vi "EngineUI.vi"() -> ()   [LabVIEW 2025, in "Abstract Engine.lvlib" / "Abstract Engine.lvclass"]
doc: "Copyright 2017 National Instruments Corporation\n\nLicensed under the Apache License, Version 2.0 (the \"License\"); you may not use this file except in compliance with the License. You may obtain a copy of the License at http://www.apache.org/licenses/LICENSE-2.0\nUnless required by applicable law or agreed to in writing, software distributed under the License is distributed on an \"AS IS\" BASIS, WITHOUT WARRANTIES OR CONDITIONS OF ANY KIND, either express or implied. See the License for the specific language governing permissions and limitations under the License."
uses:
  Abstract Engine.lvclass
  Abstract Engine.lvclass/Abstract Engine.ctl
  Engine configuration/Engine configuration.lvclass
  Users/Public/Documents/Sandia National Labs/TSS Plugin/CEF.lvlibp/Node/CEF_Node.lvclass
  <vilib>/Utility/sysdir.llb/System Directory Type.ctl
  Engine configuration/Engine Setting.ctl
  Users/Public/Documents/Sandia National Labs/TSS Plugin/CEF.lvlibp/Node/mainQref.ctl
  Users/Public/Documents/Sandia National Labs/TSS Plugin/CEF.lvlibp/Node/NodeRef.ctl
  Users/Public/Documents/Sandia National Labs/TSS Plugin/CEF.lvlibp/Node/UserEventRef.ctl
panel:
  in  "Engine Default":T1={"Enabled"=TRUE, "IP Address"="127.0.0.1", "Port"=3331, "Description"="Type = Class \n", "Type"="Engine", "Version"="1.0.0.0"}
  in  "user event":T2
  in  "main queue":T3
  in  "node ref":T4
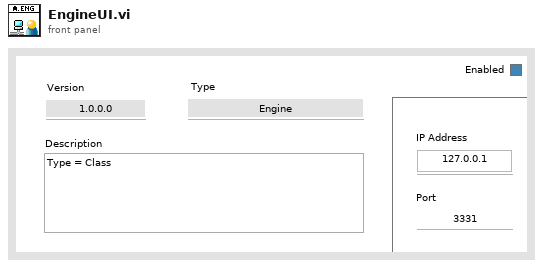
[diagram p1: front panel]
types:
  T1 = typedef "Abstract Engine.lvlib/Engine configuration.lvclass/Engine Setting.ctl" = cluster{"Enabled":bool, "IP Address":string, "Port":i32, "Description":string, "Type":string, "Version":string}
  T2 = typedef "CEF.lvlibp/CEF_Node.lvclass/UserEventRef.ctl" = refnum<user-event>
  T3 = typedef "CEF.lvlibp/CEF_Node.lvclass/mainQref.ctl" = refnum<queue>
  T4 = typedef "CEF.lvlibp/CEF_Node.lvclass/NodeRef.ctl" = refnum<data-value>
  T5 = typedef "System Directory Type.ctl" = i32
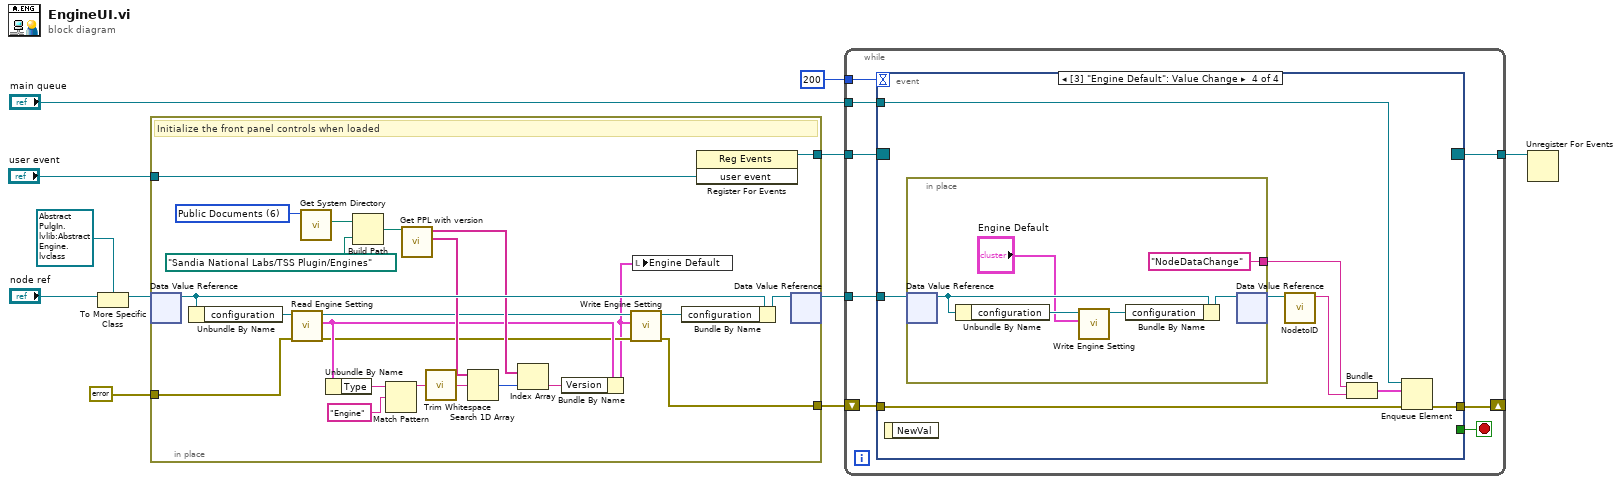
[diagram p0: block diagram]
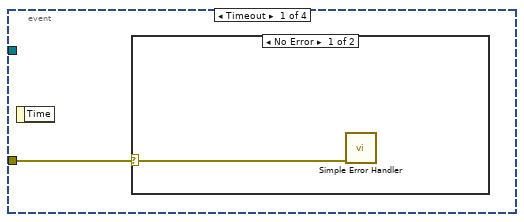
[diagram p2: hidden frame]
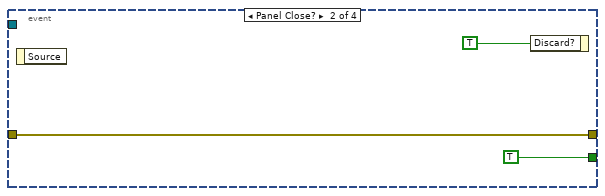
[diagram p4: hidden frame]
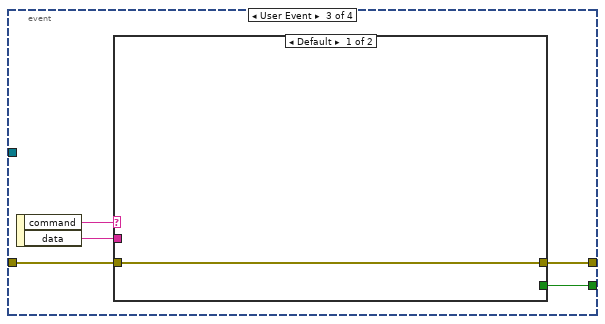
[diagram p5: hidden frame]
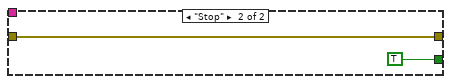
[diagram p6: hidden frame]
diagram:
  n1 = To More Specific Class(target class=refnum<data-value> refnum ("data value reference"), reference="node ref") -> (specific class reference=w7:refnum<data-value>)  [unwired: 1 in, 1 out]
  n2 = in-place {
    in-place-border: errorcluster {"status"=FALSE, "code"=0, "source"=""} ("error out") -> [w25]
    in-place-border: [w19] -> w3
    in-place-border: [w16] -> w2
    in-place-border: "user event" -> [w17]
    w31 = T5 6 items=["User Home"=0, "User Desktop"=1, "User Documents"=2, "User Application Data"=3, "User Preferences"=4, "User Temporary"=5, "Public Documents"=6, "Public Application Data"=7, "Public Preferences"=8, "Public Cache"=13, "System Core Libraries"=9, "System Installed Libraries"=10, "Application Files"=11, "Boot Volume Root"=12] ("system directory type")
    # "Initialize the front panel controls when loaded"
    n3 = in-place-dvr #1(w7) -> (w35:refnum<class "Abstract Engine.lvclass">)  [unwired: 1 out]
    n4 = Unbundle By Name(w35) -> ("configuration"=w26:refnum<class "Engine configuration.lvclass">)
    n5 = call "Read Engine Setting.vi"("error in (no error)"=w25, "Engine configuration in"=w26) -> ("error out"=w22:errorcluster, "Engine Setting"=w24:T1, "Engine configuration out"=w23:refnum<class "Engine configuration.lvclass">)  [unwired: 7 in]
    n6 = call <vilib>:"Get System Directory.vi"("system directory type"=w31) -> ("system directory"=w32:path)  [unwired: 10 in]
    n7 = Unbundle By Name(w24) -> ("Type"=w14:string)
    n8 = Build Path(base path=w32, name or relative path=path "Sandia National Labs/TSS Plugin/Engines" ("PPL folder")) -> (appended path=w30:path)
    n9 = Match Pattern(string=w14, regular expression="Engine") -> (before substring=w13:string)  [unwired: 1 in, 3 out]
    n10 = call "Get PPL with version.vi"("Plugin path"=w30) -> ("Plugin"=w29:string[], "Version"=w28:string[])  [unwired: 9 in]
    n11 = call <vilib>:"Trim Whitespace.vi"("string"=w13) -> ("trimmed string"=w12:string)  [unwired: 1 in]
    n12 = Search 1D Array(1D array=w29, element=w12) -> (index of element=w33:i32)  [unwired: 1 in]
    n13 = Index Array(array=w28, index=w33) -> (element=w27:string)
    n14 = Bundle By Name(cluster=w24, "Version"=w27) -> (w21:T1)
    n15 = call "Write Engine Setting.vi"("error in (no error)"=w22, "Engine Setting"=w21, "Engine configuration in"=w23) -> ("error out"=w19:errorcluster, "Engine configuration out"=w20:refnum<class "Engine configuration.lvclass">)  [unwired: 7 in]
    n16 = local write "Engine Default"(w21) -> ()
    n17 = Bundle By Name(cluster=w35, "configuration"=w20) -> (w34:refnum<class "Abstract Engine.lvclass">)
    n18 = register-events(w17) -> (reference out=w16:refnum<event-registration>)  [unwired: 2 in, 1 out]
    n19 = in-place-dvr #1(w34) -> (w6:refnum<data-value>)  [unwired: 1 out]
  }
  n20 = while {
    tunnel: w6 -> [w43]
    tunnel: w2 -> [w42]
    tunnel: [w41] -> w11
    tunnel: "main queue" -> [w37]
    shift-right: [w39] -> _
    shift-left: w3 -> [w38]
    tunnel: 200 -> [w36]
    stop <- w40 stop-if-true
    n21 = event shown="[3] \"Engine Default\": Value Change" {
      selector: w42 -> [_ _ _ _]
      dyn-events: [_ _ _ _] -> w41
      timeout: w36 -> [_ _ _ _]
      tunnel: w43 -> [_ _ _ w61]
      tunnel: [_ TRUE w49 _] -> w40
      tunnel: [_ w47 w50 w64] -> w39
      tunnel: w38 -> [w44 w47 w51 w60]
      tunnel: w37 -> [_ _ _ w63]
      event Timeout {
        n22 = event-data() -> ()  [unwired: 1 in, 1 out]
        n23 = case shown="No Error" w44 {
          selector: w44 -> [w45 _]
          frame No Error {
            n24 = call <vilib>:"Simple Error Handler.vi"("error in (no error)"=w45) -> ()  [unwired: 4 in, 5 out]
          }
          frame Error {
          }
        }
      }
      event Panel Close? {
        n25 = event-data() -> ()  [unwired: 1 in, 1 out]
        n26 = event-data("Discard?"=TRUE) -> ()  [unwired: 1 in, 1 out]
      }
      event User Event {
        n27 = event-data() -> ("command"=w53:string, "data"=w52:string)  [unwired: 1 in]
        n28 = case shown="Default" w53 {
          tunnel: w52 -> [_ _]
          tunnel: [_ TRUE] -> w49
          tunnel: [w54 w55] -> w50
          tunnel: w51 -> [w54 w55]
          frame Default {
          }
          frame "Stop" {
          }
        }
      }
      event Value Change {
        n29 = event-data() -> ()  [unwired: 1 in, 1 out]
        n30 = in-place {
          in-place-border: ["NodeDataChange" ("Message Name")] -> w59
          n31 = in-place-dvr #2(w61) -> (w70:refnum<class "Abstract Engine.lvclass">)  [unwired: 1 out]
          n32 = Unbundle By Name(w70) -> ("configuration"=w68:refnum<class "Engine configuration.lvclass">)
          n33 = call "Write Engine Setting.vi"("Engine Setting"="Engine Default", "Engine configuration in"=w68) -> ("Engine configuration out"=w67:refnum<class "Engine configuration.lvclass">)  [unwired: 8 in, 1 out]
          n34 = Bundle By Name(cluster=w70, "configuration"=w67) -> (w69:refnum<class "Abstract Engine.lvclass">)
          n35 = in-place-dvr #2(w69) -> (w62:refnum<data-value>)  [unwired: 1 out]
        }
        n36 = call "NodetoID.vi"("node ref"=w62) -> ("ID"=w58:string)  [unwired: 9 in, 1 out]
        n37 = Bundle("Message Name"=w59, "ID"=w58) -> (w57:cluster{"Message Name":string, "ID":string})  [unwired: 1 in]
        n38 = Enqueue Element(queue=w63, element=w57, error in (no error)=w60) -> (error out=w64:errorcluster)  [unwired: 1 in, 2 out]
      }
    }
  }
  n39 = Unregister For Events(event registration refnum=w11) -> ()  [unwired: 1 in, 1 out]
